vi "QBridge 0MQ.vi"() -> (0 "error":errorcluster)   [LabVIEW 2012]
uses:
  <vilib>/addons/zeromq/zmq_socket.lvclass
  <vilib>/addons/zeromq/socket_type.ctl
  <vilib>/addons/zeromq/socket_options.ctl
  Global_Telescopio.vi
  <vilib>/addons/zeromq/zmq_context.lvclass
  <vilib>/addons/zeromq/zeromq.lvlib
panel:
  out "focuserREP message":string
  out "Focuser160_REQ":string caption="Message to Focuser160"
  out "Focus Status":string
  in  "QueueBaseName":string="focusQueue"
  in  "stop":bool
  # "QBRIDGE ZeroMQ"
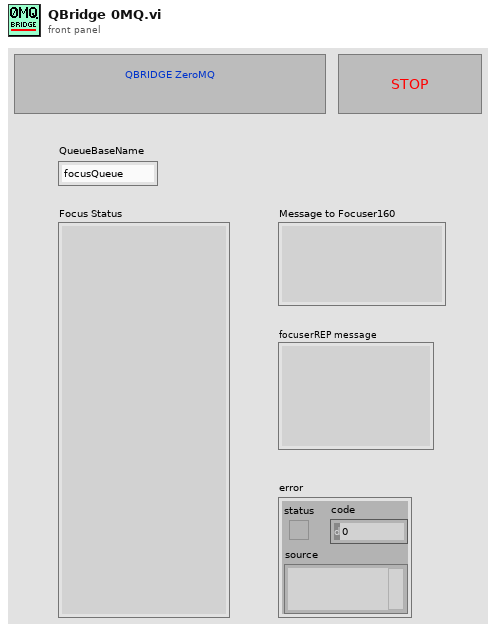
[diagram p1: front panel]
types:
  T1 = typedef "zeromq.lvlib/socket_options.ctl" = enum8{"NONE", "ZMQ_HWM", "<2>", "ZMQ_SWAP", "ZMQ_AFFINITY", "ZMQ_ROUTING_ID", "ZMQ_SUBSCRIBE", "ZMQ_UNSUBSCRIBE", "ZMQ_RATE", "ZMQ_RECOVERY_IVL", "ZMQ_MCAST_LOOP", "ZMQ_SNDBUF", "ZMQ_RCVBUF", "ZMQ_RCVMORE", "ZMQ_FD", "ZMQ_EVENTS", "ZMQ_TYPE", "ZMQ_LINGER", "ZMQ_RECONNECT_IVL", "ZMQ_BACKLOG", "ZMQ_RECOVERY_IVL_MSEC", "ZMQ_RECONNECT_IVL_MAX", "ZMQ_MAXMSGSIZE", "ZMQ_SNDHWM", "ZMQ_RCVHWM", "ZMQ_MULTICAST_HOPS", "<26>", "ZMQ_RCVTIMEO", "ZMQ_SNDTIMEO", "<29>", "<30>", "ZMQ_IPV4ONLY", "ZMQ_LAST_ENDPOINT", "ZMQ_ROUTER_MANDATORY", "ZMQ_TCP_KEEPALIVE", "ZMQ_TCP_KEEPALIVE_CNT", "ZMQ_TCP_KEEPALIVE_IDLE", "ZMQ_TCP_KEEPALIVE_INTVL", "ZMQ_TCP_ACCEPT_FILTER", "ZMQ_IMMEDIATE", "ZMQ_XPUB_VERBOSE", "ZMQ_ROUTER_RAW", "ZMQ_IPV6", "ZMQ_MECHANISM", "ZMQ_PLAIN_SERVER", "ZMQ_PLAIN_USERNAME", "ZMQ_PLAIN_PASSWORD", "ZMQ_CURVE_SERVER", "ZMQ_CURVE_PUBLICKEY", "ZMQ_CURVE_SECRETKEY", "ZMQ_CURVE_SERVERKEY", "ZMQ_PROBE_ROUTER", "ZMQ_REQ_CORRELATE", "ZMQ_REQ_RELAXED", "ZMQ_CONFLATE", "ZMQ_ZAP_DOMAIN", "ZMQ_ROUTER_HANDOVER", "ZMQ_TOS", "ZMQ_IPC_FILTER_PID", "ZMQ_IPC_FILTER_UID", "ZMQ_IPC_FILTER_GID", "ZMQ_CONNECT_ROUTING_ID", "ZMQ_GSSAPI_SERVER", "ZMQ_GSSAPI_PRINCIPAL", "ZMQ_GSSAPI_SERVICE_PRINCIPAL", "ZMQ_GSSAPI_PLAINTEXT", "ZMQ_HANDSHAKE_IVL", "<67>", "ZMQ_SOCKS_PROXY", "ZMQ_XPUB_NODROP", "ZMQ_BLOCKY", "ZMQ_XPUB_MANUAL", "ZMQ_XPUB_WELCOME_MSG", "ZMQ_STREAM_NOTIFY", "ZMQ_INVERT_MATCHING", "ZMQ_HEARTBEAT_IVL", "ZMQ_HEARTBEAT_TTL", "ZMQ_HEARTBEAT_TIMEOUT", "ZMQ_XPUB_VERBOSER", "ZMQ_CONNECT_TIMEOUT", "ZMQ_TCP_MAXRT", "ZMQ_THREAD_SAFE", "<82>", "<83>", "ZMQ_MULTICAST_MAXTPDU", "ZMQ_VMCI_BUFFER_SIZE", "ZMQ_VMCI_BUFFER_MIN_SIZE", "ZMQ_VMCI_BUFFER_MAX_SIZE", "ZMQ_VMCI_CONNECT_TIMEOUT", "ZMQ_USE_FD", "ZMQ_GSSAPI_PRINCIPAL_NAMETYPE", "ZMQ_GSSAPI_SERVICE_PRINCIPAL_NAMETYPE", "ZMQ_BINDTODEVICE", "ZMQ_ZAP_ENFORCE_DOMAIN", "ZMQ_LOOPBACK_FASTPATH", "ZMQ_METADATA", "ZMQ_MULTICAST_LOOP", "ZMQ_ROUTER_NOTIFY"}
  T2 = typedef "zeromq.lvlib/socket_type.ctl" = enum8{"ZMQ_PAIR", "ZMQ_PUB", "ZMQ_SUB", "ZMQ_REQ", "ZMQ_REP", "ZMQ_DEALER", "ZMQ_ROUTER", "ZMQ_PULL", "ZMQ_PUSH", "ZMQ_XPUB", "ZMQ_XSUB", "ZMQ_STREAM", "ZMQ_SERVER", "ZMQ_CLIENT", "ZMQ_RADIO", "ZMQ_DISH", "ZMQ_GATHER", "ZMQ_SCATTER", "ZMQ_DGRAM"}
  T3 = cluster{"broker":string, "version":string, "date":string, "hour":string, "outTemp":string, "hiTemp":string, "lowTemp":string, "outHumidity":string, "dewOut":string, "windSpeed":string, "windDirection":string, "windRun":string, "hiSpeed":string, "hiDir":string, "windChill":string, "heatIndex":string, "THWIndex":string, "THSIndex":string, "pressure":string, "rain":string, "rainRate":string, "solarRad":string, "solarEnergy":string, "hiSolarRad":string, "UVIndex":string, "UVDose":string, "hiUV":string, "headDD":string, "coolDD":string, "inTemp":string, "inHumidity":string, "inHeat":string, "inEMC":string, "inAirDensity":string, "2ndTemp":string, "2ndHumidity":string, "ET":string, "leaf":string, "windSamp":string, "windTx":string, "ISSRecept":string, "dewIn":string, "arcInt":string}
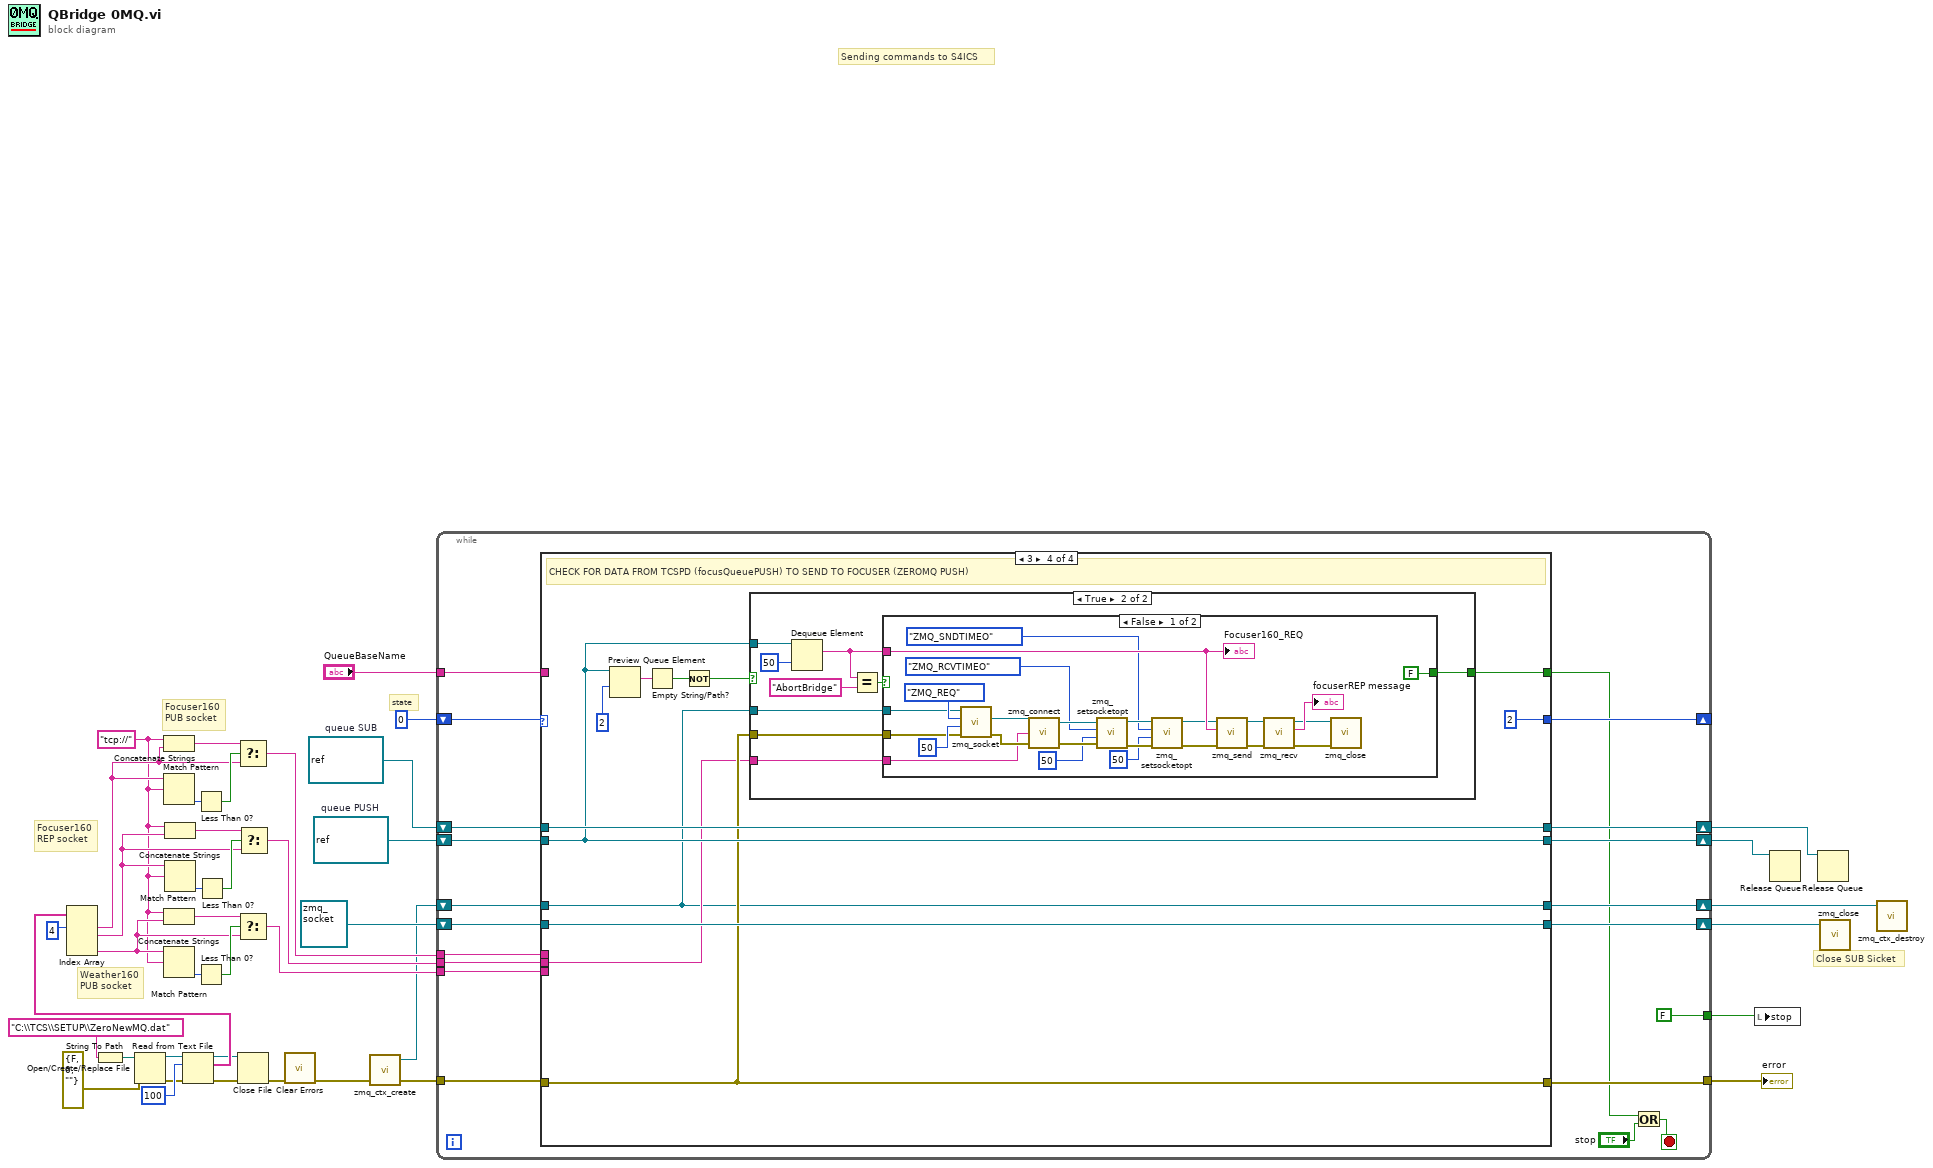
[diagram p0: block diagram]
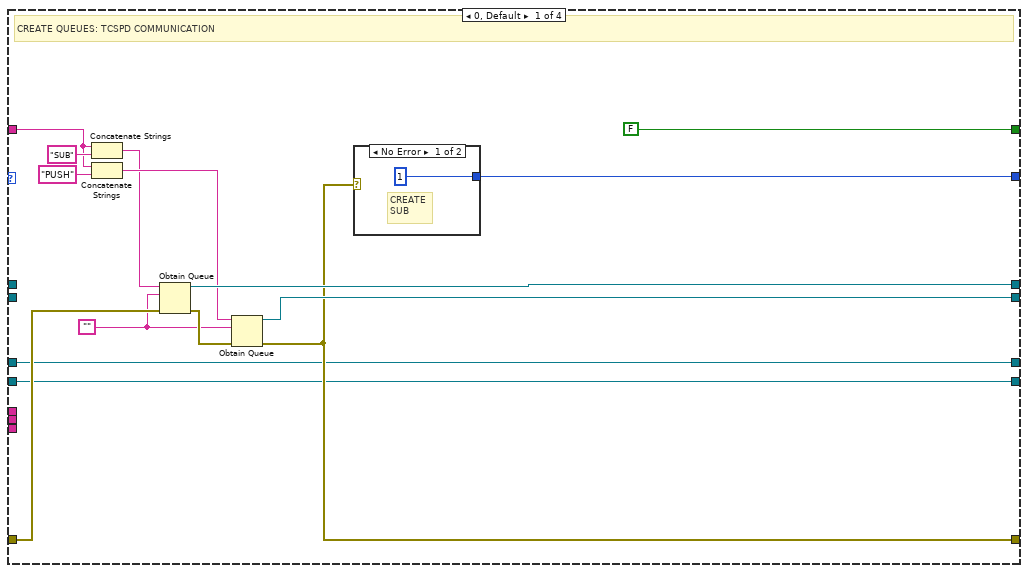
[diagram p2: hidden frame]
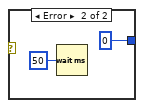
[diagram p3: hidden frame]
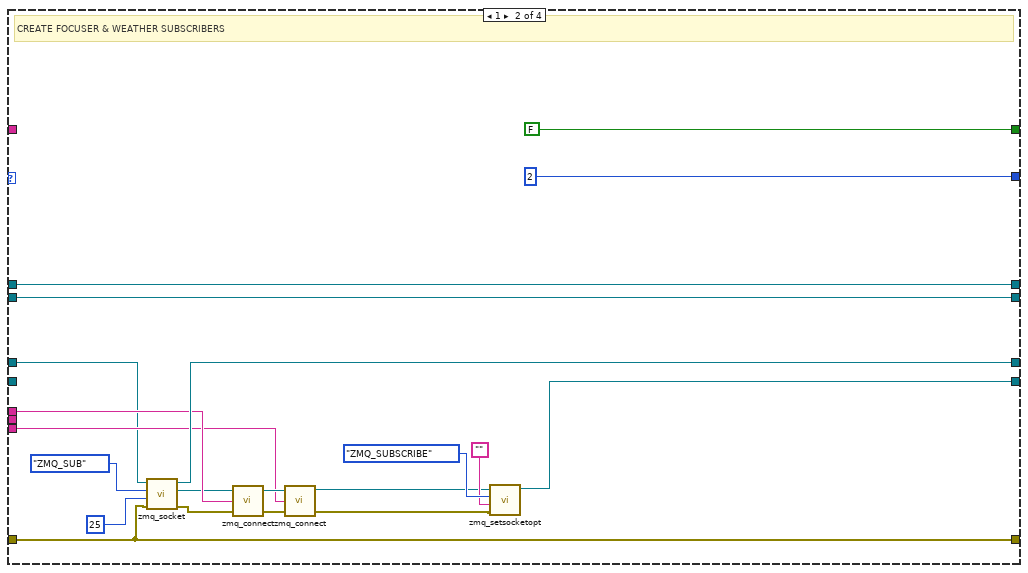
[diagram p4: hidden frame]
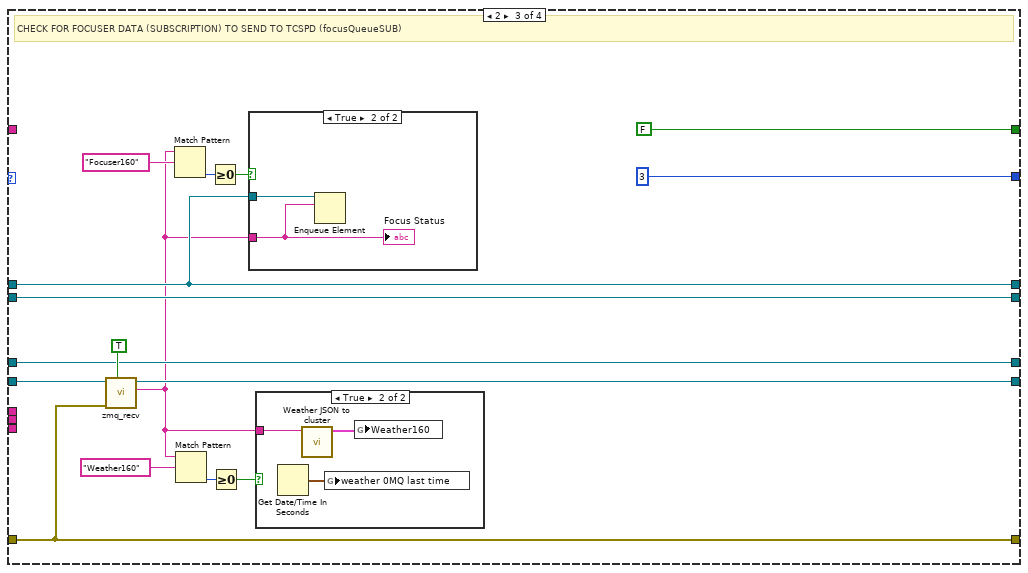
[diagram p5: hidden frame]
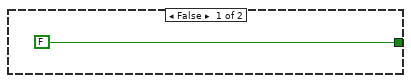
[diagram p8: hidden frame]
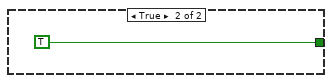
[diagram p9: hidden frame]
diagram:
  w5 = "tcp://"
  w39 = refnum<queue> refnum  # queue PUSH
  w38 = refnum<queue> refnum  # queue SUB
  # "Close SUB Sicket"
  # "Weather160\nPUB socket"
  # "Focuser160\nREP socket"
  # "Focuser160\nPUB socket"
  # "state"
  # "Sending commands to S4ICS"
  n1 = String To Path(string="C:\\TCS\\SETUP\\ZeroNewMQ.dat") -> (path=w36:path)
  n2 = Open/Create/Replace File(file path (use dialog)=w36, error in=errorcluster {"status"=FALSE, "code"=0, "source"=""}) -> (refnum out=w34:refnum<file>, error out=w27:errorcluster)  [unwired: 4 in, 1 out]
  n3 = Read from Text File(file (use dialog)=w34, count=100, error in=w27) -> (refnum out=w30:refnum<file>, text=w32:string[], error out=w22:errorcluster)  [unwired: 1 in, 1 out]
  n4 = Index Array(array=w32, index #1=4 ("index")) -> (element #1=w11:string, element #2=w16:string, element #4=w6:string)  [unwired: 3 in, 1 out]
  n5 = Concatenate Strings(w5, w11) -> (w13:string)
  n6 = Match Pattern(string=w11, regular expression=w5) -> (offset past match=w12:i32)  [unwired: 1 in, 3 out]
  n7 = Concatenate Strings(w5, w6) -> (w8:string)
  n8 = Match Pattern(string=w6, regular expression=w5) -> (offset past match=w9:i32)  [unwired: 1 in, 3 out]
  n9 = Concatenate Strings(w5, w16) -> (w18:string)
  n10 = Match Pattern(string=w16, regular expression=w5) -> (offset past match=w17:i32)  [unwired: 1 in, 3 out]
  n11 = Less Than 0?(x=w12) -> (x < 0?=w14:bool)
  n12 = Less Than 0?(x=w9) -> (x < 0?=w7:bool)
  n13 = Less Than 0?(x=w17) -> (x < 0?=w19:bool)
  n14 = Select(t=w13, s=w14, f=w11) -> (s? t:f=w10:string)
  n15 = Select(t=w8, s=w7, f=w6) -> (s? t:f=w4:string)
  n16 = Close File(refnum=w30, error in=w22) -> (error out=w23:errorcluster)  [unwired: 1 out]
  n17 = Select(t=w18, s=w19, f=w16) -> (s? t:f=w15:string)
  n18 = call <vilib>:"Clear Errors.vi"("error in (no error)"=w23) -> ("error out"=w3:errorcluster)  [unwired: 6 in]
  n19 = call <vilib>:"zmq_ctx_create.vi"("error in"=w3) -> ("error out"=w2:errorcluster, "context out"=w1:refnum<class "zmq_context.lvclass">)  [unwired: 3 in]
  n20 = while {
    shift-right: [w59] -> _
    shift-left: u16 0 -> [w61]
    shift-right: [w55] -> w25
    shift-left: w38 -> [w53]
    shift-right: [w54] -> w24
    shift-left: w39 -> [w52]
    tunnel: w2 -> [w60]
    tunnel: [w58] -> w40
    tunnel: "QueueBaseName" -> [w51]
    tunnel: w10 -> [w50]
    tunnel: w15 -> [w49]
    shift-right: [w47] -> w21
    shift-left: refnum<class "zmq_socket.lvclass"> refnum ("socket out") -> [w48]
    shift-right: [w46] -> w26
    shift-left: w1 -> [w44]
    tunnel: [FALSE] -> w20
    tunnel: w4 -> [w42]
    stop <- w56 stop-if-true
    n21 = case shown="3" w61 {
      tunnel: w60 -> [w73 w80 w107 w126]
      tunnel: [w74 u16 2 u16 3 u16 2] -> w59
      tunnel: [w71 w80 w107 w126] -> w58
      tunnel: [w76 w98 w112 w132] -> w55
      tunnel: [w75 w97 w115 w128] -> w54
      tunnel: w53 -> [_ w98 w112 w132]
      tunnel: w52 -> [_ w97 w115 w128]
      tunnel: w51 -> [w65 _ _ _]
      tunnel: w50 -> [_ w94 _ _]
      tunnel: w49 -> [_ _ _ w122]
      tunnel: w48 -> [w64 _ w114 w127]
      tunnel: [w64 w99 w113 w127] -> w47
      tunnel: [w62 w96 w108 w121] -> w46
      tunnel: [FALSE FALSE FALSE w124] -> w45
      tunnel: w44 -> [w62 w81 w108 w121]
      tunnel: w42 -> [_ w84 _ _]
      frame 0, Default {
        w66 = ""
        # "CREATE QUEUES: TCSPD COMMUNICATION"
        n22 = Concatenate Strings(w65, "SUB" ("string")) -> (w67:string)
        n23 = Concatenate Strings(w65, "PUSH" ("string")) -> (w69:string)
        n24 = Obtain Queue(name (unnamed)=w67, element data type=w66, error in (no error)=w73) -> (queue out=w76:refnum<queue>, error out=w72:errorcluster)  [unwired: 2 in, 1 out]
        n25 = Obtain Queue(name (unnamed)=w69, element data type=w66, error in (no error)=w72) -> (queue out=w75:refnum<queue>, error out=w71:errorcluster)  [unwired: 2 in, 1 out]
        n26 = case shown="No Error" w71 {
          tunnel: [u16 1 u16 0] -> w74
          frame No Error {
            # "CREATE\nSUB"
          }
          frame Error {
            n27 = Wait (ms)(milliseconds to wait=u32 50) -> ()  [unwired: 1 out]
          }
        }
      }
      frame 1 {
        # "CREATE FOCUSER & WEATHER SUBSCRIBERS"
        n28 = call <vilib>:"zmq_socket.vi"("error in"=w80, "linger (ms)"=25, "socket type"=socket_type."ZMQ_SUB", "context in"=w81) -> ("error out"=w91:errorcluster, "socket out"=w92:refnum<class "zmq_socket.lvclass">, "context out"=w96:refnum<class "zmq_context.lvclass">)  [unwired: 1 in]
        n29 = call <vilib>:"zmq_connect.vi"("error in"=w91, "endpoint"=w94, "socket in"=w92) -> ("error out"=w85:errorcluster, "socket out"=w86:refnum<class "zmq_socket.lvclass">)  [unwired: 1 in]
        n30 = call <vilib>:"zmq_connect.vi"("error in"=w85, "endpoint"=w84, "socket in"=w86) -> ("error out"=w83:errorcluster, "socket out"=w82:refnum<class "zmq_socket.lvclass">)  [unwired: 1 in]
        n31 = call <vilib>:"zmq_setsocketopt.vi"("error in"=w83, "value"="", "option"=socket_options."ZMQ_SUBSCRIBE", "socket in"=w82) -> ("socket out"=w99:refnum<class "zmq_socket.lvclass">)  [unwired: 2 in, 1 out]
      }
      frame 2 {
        # "CHECK FOR FOCUSER DATA (SUBSCRIPTION) TO SEND TO TCSPD (focusQueueSUB)"
        n32 = call <vilib>:"zmq_recv.vi"("no block? (F)"=TRUE, "error in"=w107, "socket in"=w114) -> ("data"=w100:string, "socket out"=w113:refnum<class "zmq_socket.lvclass">)  [unwired: 2 in, 3 out]
        n33 = Match Pattern(string=w100, regular expression="Focuser160") -> (offset past match=w106:i32)  [unwired: 1 in, 3 out]
        n34 = Match Pattern(string=w100, regular expression="Weather160") -> (offset past match=w102:i32)  [unwired: 1 in, 3 out]
        n35 = Greater Or Equal To 0?(x=w106) -> (x >= 0?=w105:bool)
        n36 = Greater Or Equal To 0?(x=w102) -> (x >= 0?=w101:bool)
        n37 = case shown="True" w105 {
          tunnel: w112 -> [_ w120]
          tunnel: w100 -> [_ w119]
          frame False {
          }
          frame True {
            n38 = Enqueue Element(queue=w120, element=w119) -> ()  [unwired: 2 in, 3 out]
            "Focus Status" <- w119
          }
        }
        n39 = case shown="True" w101 {
          tunnel: w100 -> [_ w118]
          frame False {
          }
          frame True {
            n40 = Get Date/Time In Seconds() -> (seconds since 1Jan1904=w117:timestamp)
            n41 = call "Weather JSON to cluster.vi"("JSON status"=w118) -> ("Weather160"=w116:T3)  [unwired: 10 in]
            n42 = global write "Global_Telescopio.vi" "weather 0MQ last time"(w117) -> ()
            n43 = global write "Global_Telescopio.vi" "Weather160"(w116) -> ()
          }
        }
      }
      frame 3 {
        # "CHECK FOR DATA FROM TCSPD (focusQueuePUSH) TO SEND TO FOCUSER (ZEROMQ PUSH)"
        n44 = Preview Queue Element(queue=w128, timeout in ms (-1)=2) -> (element=w131:string)  [unwired: 1 in, 3 out]
        n45 = Empty String/Path?(string/path=w131) -> (empty?=w130:bool)
        n46 = Not(x=w130) -> (.not. x?=w129:bool)
        n47 = case shown="True" w129 {
          tunnel: w128 -> [_ w142]
          tunnel: w122 -> [_ w140]
          tunnel: w126 -> [_ w141]
          tunnel: [FALSE w136] -> w124
          tunnel: w121 -> [_ w134]
          frame False {
          }
          frame True {
            n48 = Dequeue Element(queue=w142, timeout in ms (-1)=50) -> (element=w138:string)  [unwired: 1 in, 3 out]
            n49 = Equal?(x=w138, y="AbortBridge") -> (x = y?=w137:bool)
            n50 = case shown="False" w137 {
              tunnel: w141 -> [w159 _]
              tunnel: w140 -> [w164 _]
              tunnel: w138 -> [w163 _]
              tunnel: [FALSE TRUE] -> w136
              tunnel: w134 -> [w158 _]
              frame False {
                n51 = call <vilib>:"zmq_socket.vi"("error in"=w159, "linger (ms)"=50, "socket type"=socket_type."ZMQ_REQ", "context in"=w158) -> ("error out"=w166:errorcluster, "socket out"=w165:refnum<class "zmq_socket.lvclass">)  [unwired: 1 in, 1 out]
                n52 = call <vilib>:"zmq_connect.vi"("error in"=w166, "endpoint"=w164, "socket in"=w165) -> ("error out"=w152:errorcluster, "socket out"=w151:refnum<class "zmq_socket.lvclass">)  [unwired: 1 in]
                n53 = call <vilib>:"zmq_setsocketopt.vi"("error in"=w152, "value"=50 ("linger (ms)"), "option"=socket_options."ZMQ_RCVTIMEO", "socket in"=w151) -> ("error out"=w149:errorcluster, "socket out"=w148:refnum<class "zmq_socket.lvclass">)  [unwired: 2 in]
                n54 = call <vilib>:"zmq_setsocketopt.vi"("error in"=w149, "value"=50 ("linger (ms)"), "option"=socket_options."ZMQ_SNDTIMEO", "socket in"=w148) -> ("error out"=w144:errorcluster, "socket out"=w143:refnum<class "zmq_socket.lvclass">)  [unwired: 2 in]
                n55 = call <vilib>:"zmq_send.vi"("error in"=w144, "data"=w163, "socket in"=w143) -> ("error out"=w157:errorcluster, "socket out"=w156:refnum<class "zmq_socket.lvclass">)  [unwired: 4 in]
                n56 = call <vilib>:"zmq_recv.vi"("error in"=w157, "socket in"=w156) -> ("error out"=w153:errorcluster, "data"=→"focuserREP message":string, "socket out"=w154:refnum<class "zmq_socket.lvclass">)  [unwired: 3 in, 2 out]
                n57 = call <vilib>:"zmq_close.vi"("error in"=w153, "socket"=w154) -> ()  [unwired: 3 in, 1 out]
                "Focuser160_REQ" <- w163
              }
              frame True {
              }
            }
          }
        }
      }
    }
    n58 = Or(x=w45, y="stop") -> (x .or. y?=w56:bool)
  }
  "error" <- w40
  n59 = local write "stop"(w20) -> ()
  n60 = Release Queue(queue=w24) -> ()  [unwired: 2 in, 3 out]
  n61 = Release Queue(queue=w25) -> ()  [unwired: 2 in, 3 out]
  n62 = call <vilib>:"zmq_close.vi"("socket"=w21) -> ()  [unwired: 4 in, 1 out]
  n63 = call <vilib>:"zmq_ctx_destroy.vi"("context in"=w26) -> ()  [unwired: 4 in, 1 out]
